vi "getAll.vi"(8 "error in (no error)":errorcluster, 11 "instrument.PPMS2 in":refnum<class "instrument.PPMS.lvclass">) -> (0 "error out":errorcluster, 2 "getAll":variant, 3 "instrument.PPMS2 out":refnum<class "instrument.PPMS.lvclass">)   [LabVIEW 2016, in "instrument.PPMS.lvclass"]
uses:
  instrument.PPMS.lvclass
  Typedefs/getAll--PPMS--cluster.ctl
  Typedefs/Temperature Status--PPMS--ring.ctl
  Typedefs/Magnet Status--PPMS--ring.ctl
  instrument.PPMS.lvclass/instrument.PPMS.ctl
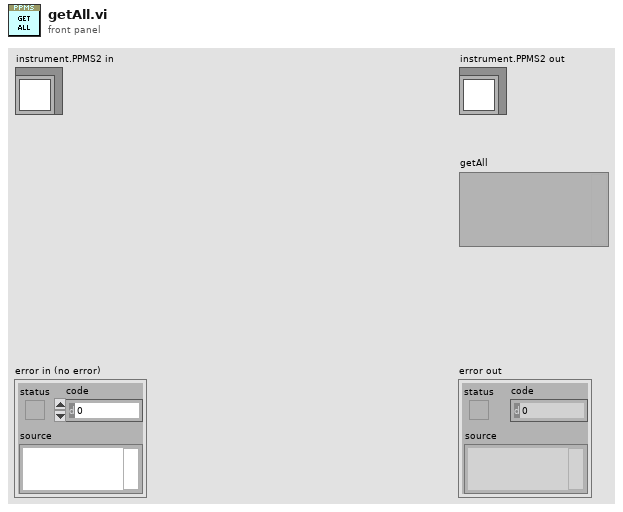
[diagram p1: front panel]
types:
  T1 = typedef "instrument.PPMS.lvclass/getAll--PPMS--cluster.ctl" = cluster{"PPMS 1 Helium Level":dbl, "PPMS 1 Temperature":dbl, "PPMS 1 Temperature Status":T2, "PPMS 1 Magnetic Field":dbl, "PPMS 1 Magnet Status":T3}
  T2 = typedef "instrument.PPMS.lvclass/Temperature Status--PPMS--ring.ctl" = i32
  T3 = typedef "instrument.PPMS.lvclass/Magnet Status--PPMS--ring.ctl" = i32
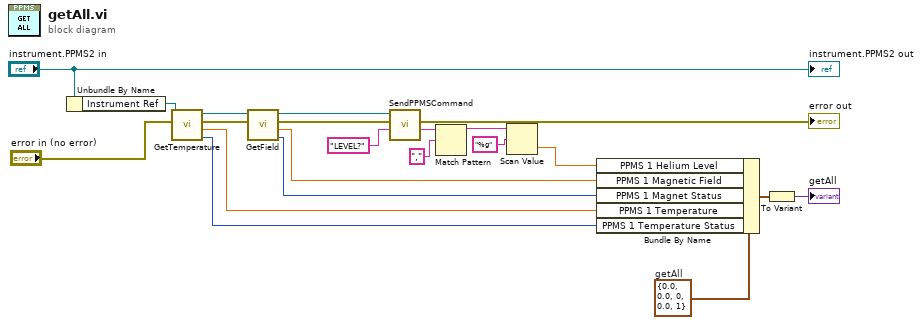
[diagram p0: block diagram]
diagram:
  w13 = T1 {"PPMS 1 Helium Level"=0.0, "PPMS 1 Temperature"=0.0, "PPMS 1 Temperature Status"=0, "PPMS 1 Magnetic Field"=0.0, "PPMS 1 Magnet Status"=1}  # getAll
  n1 = Unbundle By Name("instrument.PPMS2 in") -> ("Instrument Ref"=w7:refnum<k24>)
  n2 = call "GetTemperature.vi"("error in (no error)"="error in (no error)", "Instrument Ref In"=w7) -> ("Temperature\nStatus"=w2:i32, "Temperature"=w11:dbl, "error out"=w20:errorcluster, "Instrument Ref Out"=w19:refnum<k24>)  [unwired: 3 in, 1 out]
  n3 = call "GetField.vi"("error in (no error)"=w20, "Instrument Ref In"=w19) -> ("Field\nStatus"=w3:i32, "Field"=w12:dbl, "error out"=w17:errorcluster, "Instrument Ref Out"=w18:refnum<k24>)  [unwired: 3 in, 1 out]
  n4 = call "SendPPMSCommand.vi"("PpmsCommand"="LEVEL?", "error in (no error)"=w17, "Instrument Ref In"=w18) -> ("PpmsReply"=w21:string, "error out"=→"error out":errorcluster)  [unwired: 4 in, 3 out]
  n5 = Match Pattern(string=w21, regular expression=",") -> (before substring=w10:string)  [unwired: 1 in, 3 out]
  n6 = Scan Value(string=w10, format string="%g") -> (value=w1:dbl)  [unwired: 1 in, 1 out]
  n7 = Bundle By Name(cluster=w13, "PPMS 1 Helium Level"=w1, "PPMS 1 Magnetic Field"=w12, "PPMS 1 Magnet Status"=w3, "PPMS 1 Temperature"=w11, "PPMS 1 Temperature Status"=w2) -> (w4:T1)
  n8 = To Variant(anything=w4) -> (Variant=→"getAll":variant)
  "instrument.PPMS2 out" <- "instrument.PPMS2 in"
